vi "check_uncheck_list.vi"(8 "error in (no error)":errorcluster, 10 "Coords":T1, 11 "MulticolumnListbox in":refnum<vi>) -> (0 "error out":errorcluster, 3 "ItemSyms":i32[](array[numeric]))   [LabVIEW 2020, in "lv_documentation.lvlib"]
uses:
  lv_documentation.lvlib
  <vilib>/Utility/miscctls.llb/LVPoint32TypeDef.ctl
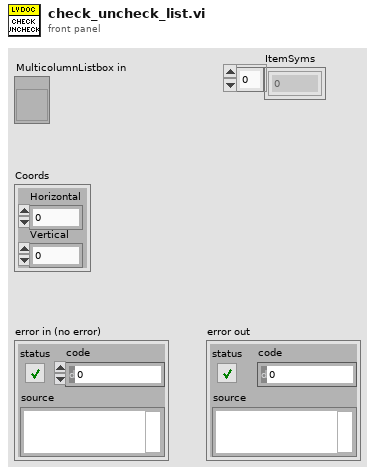
[diagram p1: front panel]
types:
  T1 = typedef "LVPoint32TypeDef.ctl" = cluster{"Horizontal":i32, "Vertical":i32}
  T2 = typedef "LVRowAndColumnTypeDef.ctl" = cluster{"Row":i32, "Column":i32}
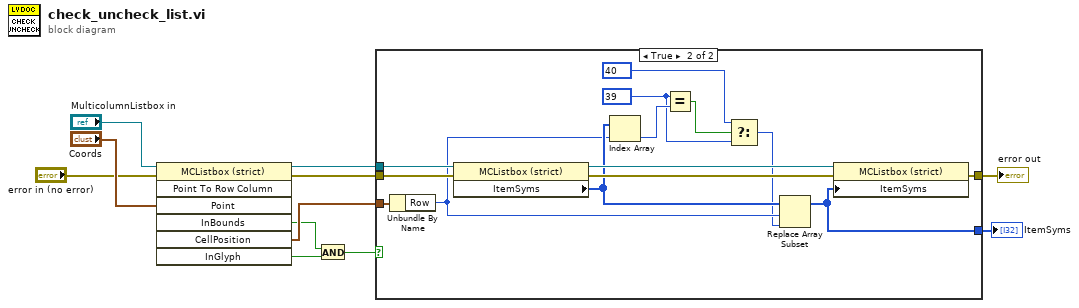
[diagram p0: block diagram]
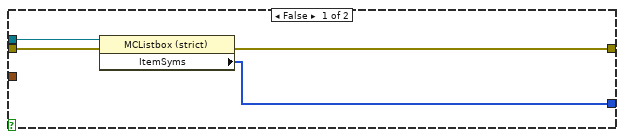
[diagram p2: hidden frame]
diagram:
  n1 = invoke class="MCListbox (strict)" method="Point To Row Column"(reference="MulticolumnListbox in", error in="error in (no error)", "Point"="Coords") -> (reference out=w9:refnum<vi>, error out=w3:errorcluster, "InBounds"=w6:bool, "CellPosition"=w8:T2, "InGlyph"=w7:bool)  [unwired: 4 in, 2 out]
  n2 = And(x=w6, y=w7) -> (x .and. y?=w11:bool)
  n3 = case shown="True" w11 {
    tunnel: w3 -> [w14 w29]
    tunnel: w8 -> [_ w28]
    tunnel: w9 -> [w15 w26]
    tunnel: [w13 w25] -> w10
    tunnel: [w12 w16] -> w1
    frame False {
      n4 = property class="MCListbox (strict)"(reference=w15, error in=w14) -> (error out=w13:errorcluster, "ItemSyms"=w12:i32[])  [unwired: 1 out]
    }
    frame True {
      w21 = 39
      n5 = Unbundle By Name(w28) -> ("Row"=w18:i32)
      n6 = property class="MCListbox (strict)"(reference=w26, error in=w29) -> (reference out=w24:refnum<vi>, error out=w27:errorcluster, "ItemSyms"=w19:i32[])
      n7 = Index Array(array=w19, index=w18) -> (element=w23:i32)
      n8 = Equal?(x=w21, y=w23) -> (x = y?=w22:bool)
      n9 = Select(t=40, s=w22, f=w21) -> (s? t:f=w17:i32)
      n10 = Replace Array Subset(array=w19, new element=w17, index=w18) -> (w16:i32[])
      n11 = property class="MCListbox (strict)"(reference=w24, error in=w27, "ItemSyms"=w16) -> (error out=w25:errorcluster)  [unwired: 1 out]
    }
  }
  "error out" <- w10
  "ItemSyms" <- w1
